vi "QueryServer_Stop.vi"(0 "Server Info":T2, 2 "Event Registration Refnum":refnum<event-registration>, 3 "error in (no error)":errorcluster) -> (10 "error out":errorcluster)   [LabVIEW 2019, in "labview-grpc-query-server.lvlib"]
uses:
  labview-grpc-query-server.lvlib
  QueryServer_InvokeEventData.ctl
  gRPC interface/Server API/typeDefs/grpcId.ctl
  gRPC interface/gprc-lvsupport.lvlib
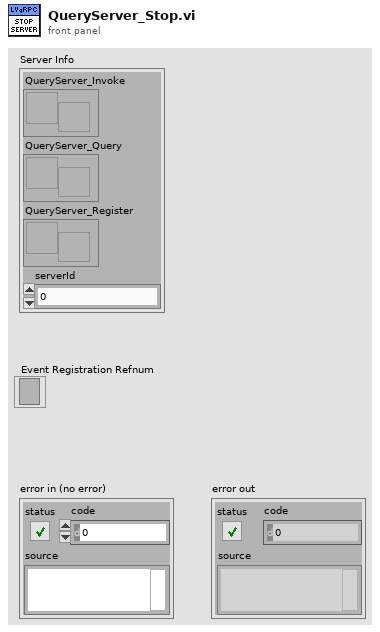
[diagram p1: front panel]
types:
  T1 = typedef "gprc-lvsupport.lvlib/grpcId.ctl" = u64
  T2 = cluster{"QueryServer_Invoke":refnum<user-event>, "QueryServer_Query":refnum<user-event>, "QueryServer_Register":refnum<user-event>, "serverId":T1}
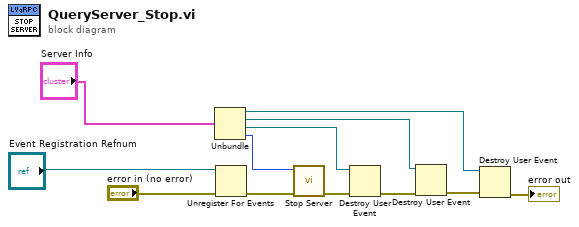
[diagram p0: block diagram]
diagram:
  n1 = Unbundle("Server Info") -> ("QueryServer_Invoke"=w6:refnum<user-event>, "QueryServer_Query"=w7:refnum<user-event>, "QueryServer_Register"=w8:refnum<user-event>, "serverId"=w2:T1)
  n2 = Unregister For Events(event registration refnum="Event Registration Refnum", error in="error in (no error)") -> (error out=w4:errorcluster)
  n3 = call "Stop Server.vi"("error in (no error)"=w4, "Server Id"=w2) -> ("error out"=w3:errorcluster)  [unwired: 9 in]
  n4 = Destroy User Event(user event=w8, error in=w3) -> (error out=w11:errorcluster)
  n5 = Destroy User Event(user event=w7, error in=w11) -> (error out=w10:errorcluster)
  n6 = Destroy User Event(user event=w6, error in=w10) -> (error out=→"error out":errorcluster)
